vi "Host_Main.vi"() -> ()   [LabVIEW 2019]
uses:
  <vilib>/vision/NI_Vision_Development_Module.lvlib
panel:
  in  "stop":bool
  out "HeartBeatSignal":bool
  out "ZMP_Y-Axis_Position(mm)":dbl format="%.1f"
  out "XY Graph":cluster{dbl[], dbl[]}[](graph)
  out "ZMP_X-Axis_Position(mm)":dbl format="%.1f"
  in  "Ladeer_Mass(Kg)":dbl=1000.0
  in  "Ladeer_Mass_Point(mm)":dbl=1000.0
  in  "Load(Kg)":dbl=100.0
  in  "Outrigger_Front_Position(mm)":dbl=1500.0
  in  "Outrigger_Rear_Position(mm)":dbl=100.0
  in  "Outrigger_RR_Length(mm)":dbl=300.0
  in  "Outrigger_RL_Length(mm)":dbl=-300.0
  in  "Outrigger_FR_Length(mm)":dbl=500.0
  in  "Outrigger_FL_Length(mm)":dbl=-500.0
  in  "Vehicle_Mass(Kg)":dbl
  in  "Boom_Rising_Angle(Degree)":dbl
  in  "Boom_Rotation_Angle(Degree)":dbl
  # "Aerial Ladder Truck Monitoring Program"
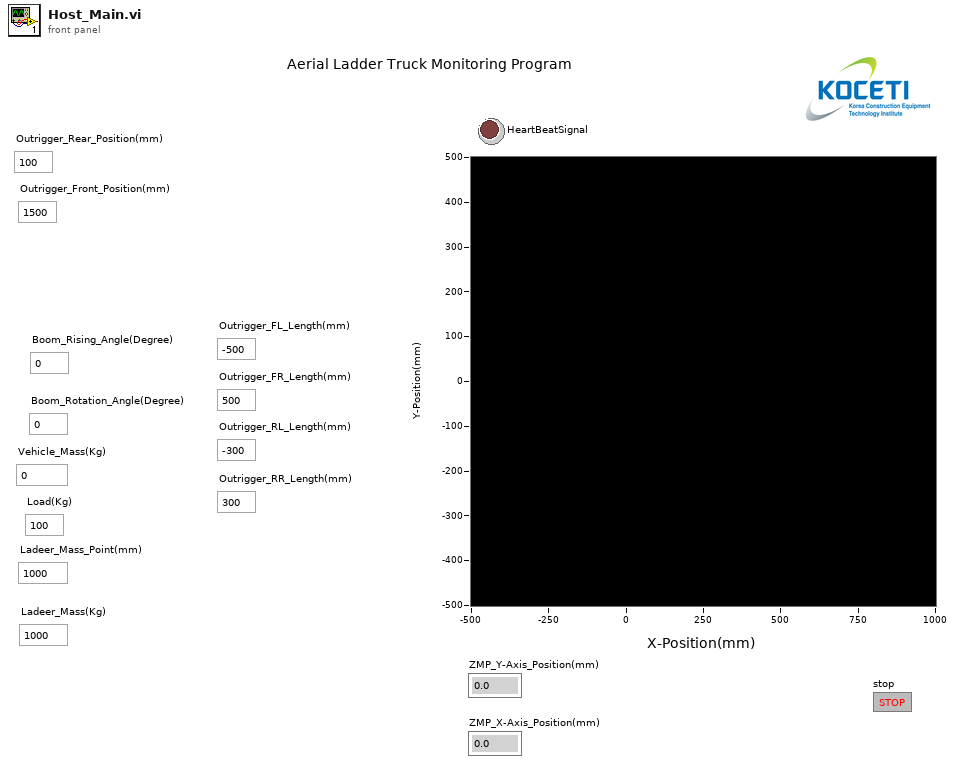
[diagram p1: front panel]
types:
  T1 = cluster{"Red or Hue value":u8, "Green or Sat value":u8, "Blue or Luma or Val or Inten value":u8}
  T2 = typedef "Image Type" = u32
  T3 = typedef "IMAQ Image.ctl" = refnum<image>
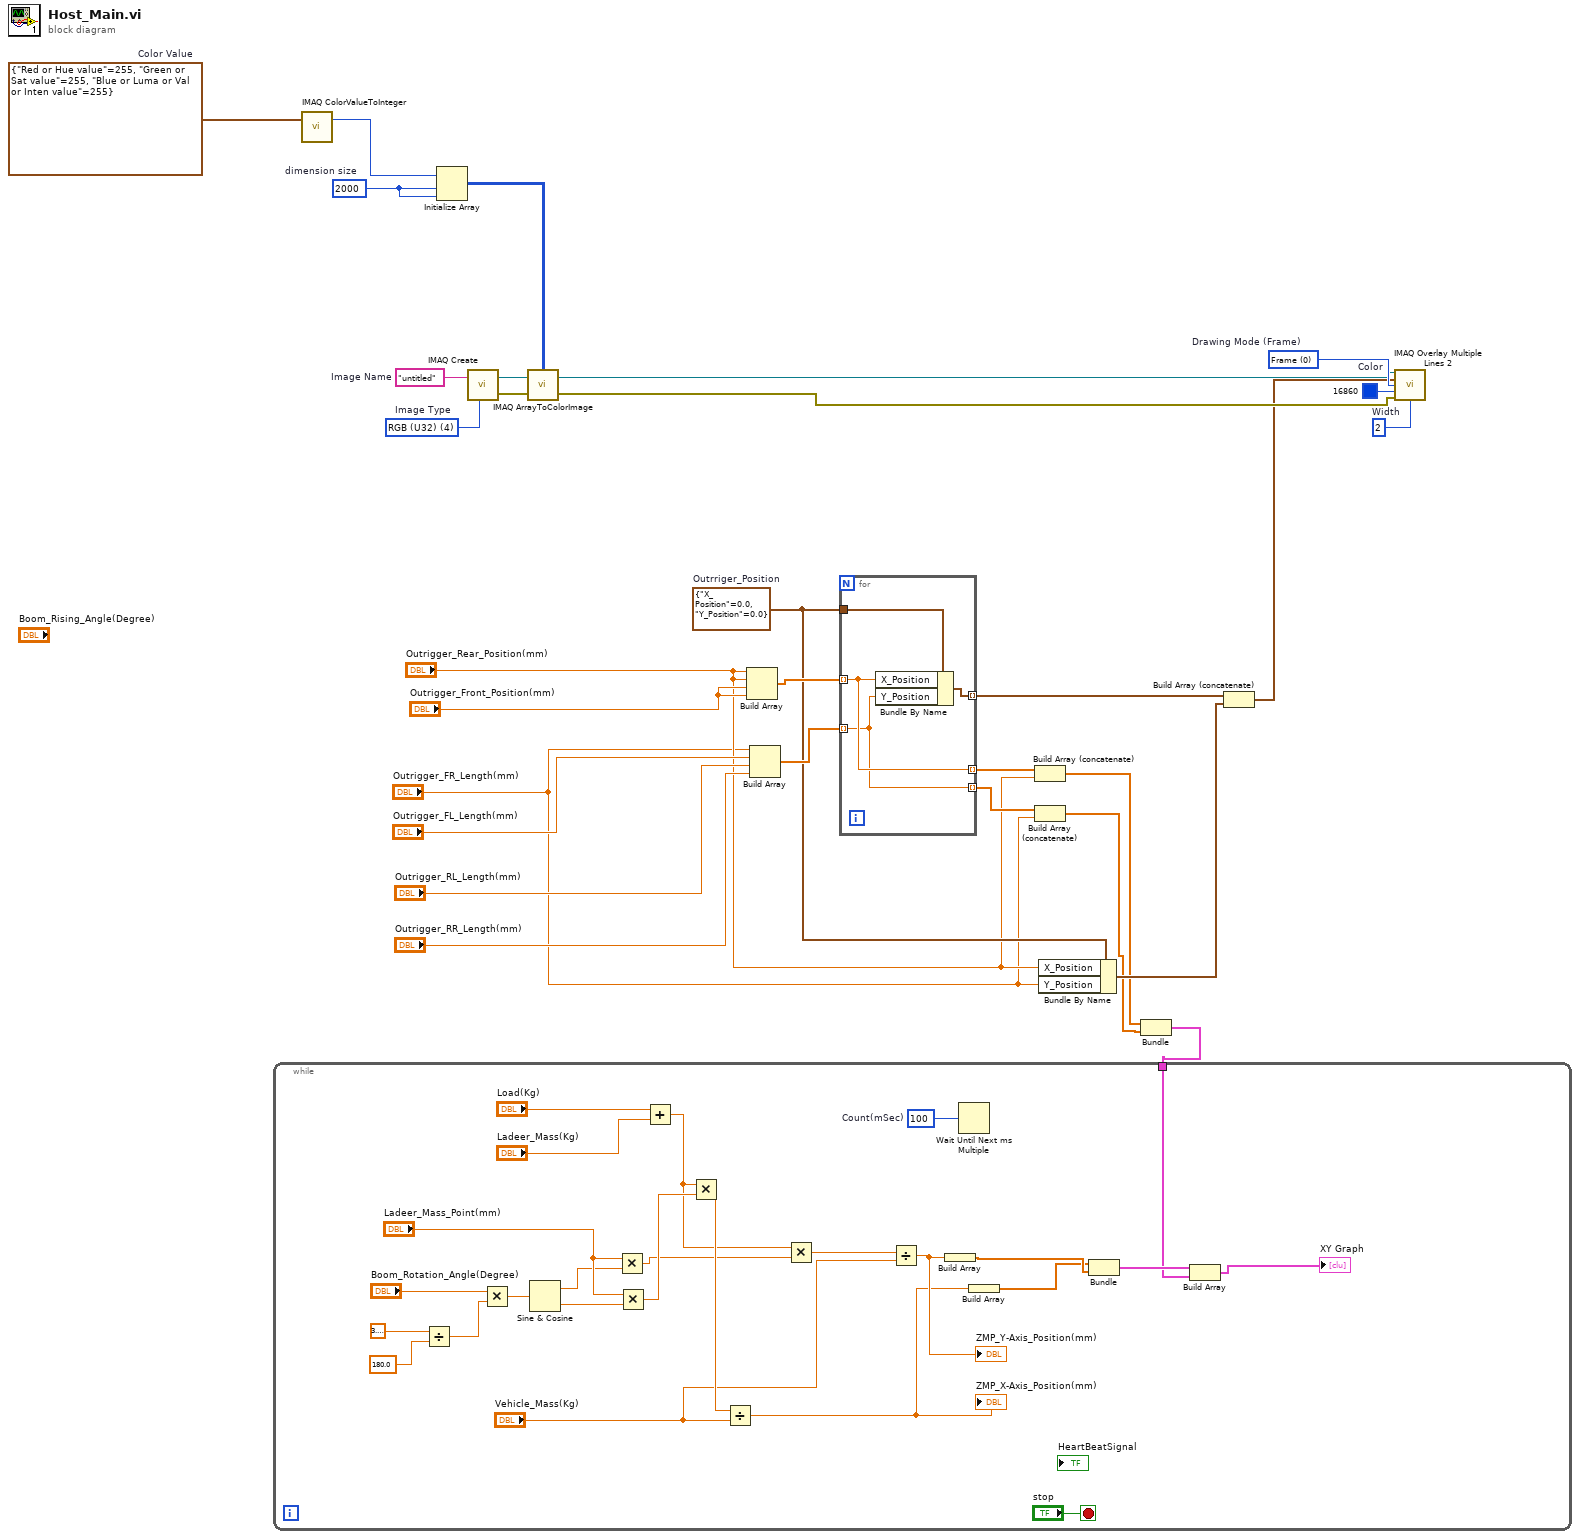
[diagram p0: block diagram]
diagram:
  w14 = 2000  # dimension size
  w18 = T1 {"Red or Hue value"=255, "Green or Sat value"=255, "Blue or Luma or Val or Inten value"=255}  # Color Value
  w20 = u32 2  # Width
  w21 = u32 0 items=["Frame", "Fill"]  # Drawing Mode (Frame)
  w22 = T2 4 items=["Grayscale (U8)", "Grayscale (I16)", "Grayscale (SGL)", "Complex (CSG)", "RGB (U32)", "HSL (U32)", "RGB (U64)", "Grayscale (U16)"]  # Image Type
  w23 = "untitled"  # Image Name
  w24 = u32 16860  # Color
  w11 = cluster{"X_Position":dbl, "Y_Position":dbl} {"X_Position"=0.0, "Y_Position"=0.0}  # Outrriger_Position
  n1 = call "IMAQ ColorValueToInteger"("Color Value"=w18) -> ("U32 value"=w16:u32)  [unwired: 4 in, 3 out]
  n2 = Initialize Array "Initialize Array"(w16, w14, w14) -> (w15:u32[][])
  n3 = call "IMAQ Create"("Image Name"=w23, "Image Type"=w22) -> ("New Image"=w19:T3, "error out"=w10:errorcluster)  [unwired: 3 in]
  n4 = call "IMAQ ArrayToColorImage"("Image Pixels (U32)"=w15, "Image"=w19, "error in (no error)"=w10) -> ("Image Out"=w17:T3, "error out"=w9:errorcluster)  [unwired: 2 in]
  n5 = Build Array("Outrigger_Rear_Position(mm)", "Outrigger_Rear_Position(mm)", "Outrigger_Front_Position(mm)", "Outrigger_Front_Position(mm)") -> (w30:dbl[])
  n6 = Build Array("Outrigger_FR_Length(mm)", "Outrigger_FL_Length(mm)", "Outrigger_RL_Length(mm)", "Outrigger_RR_Length(mm)") -> (w29:dbl[])
  n7 = for {
    tunnel: w30 -> [w32] mode=indexing
    tunnel: w11 -> [w34]
    tunnel: w29 -> [w31] mode=indexing
    tunnel: [w33] -> w25 mode=indexing
    tunnel: [w32] -> w8 mode=indexing
    tunnel: [w31] -> w7 mode=indexing
    n8 = Bundle By Name(cluster=w34, "X_Position"=w32, "Y_Position"=w31) -> (w33:cluster{"X_Position":dbl, "Y_Position":dbl})
  }
  n9 = Build Array (concatenate)(w8, "Outrigger_Rear_Position(mm)") -> (w4:dbl[])
  n10 = Build Array (concatenate)(w7, "Outrigger_FR_Length(mm)") -> (w3:dbl[])
  n11 = Bundle By Name(cluster=w11, "X_Position"="Outrigger_Rear_Position(mm)", "Y_Position"="Outrigger_FR_Length(mm)") -> (w12:cluster{"X_Position":dbl, "Y_Position":dbl})
  n12 = Bundle(w4, w3) -> (w2:cluster{dbl[], dbl[]})  [unwired: 1 in]
  n13 = while {
    tunnel: w2 -> [w36]
    stop <- "stop" stop-if-true
    w49 = u32 100  # Count(mSec)
    n14 = Divide(x=3.141592653589793, y=180.0) -> (x/y=w56:dbl)
    n15 = Multiply(x="Boom_Rotation_Angle(Degree)", y=w56) -> (x*y=w57:dbl)
    n16 = Sine & Cosine(0:w57) -> (1:w46:dbl, 2:w51:dbl)
    n17 = Multiply(x="Ladeer_Mass_Point(mm)", y=w46) -> (x*y=w45:dbl)
    n18 = Multiply(x="Ladeer_Mass_Point(mm)", y=w51) -> (x*y=w50:dbl)
    n19 = Add(x="Load(Kg)", y="Ladeer_Mass(Kg)") -> (x+y=w48:dbl)
    n20 = Multiply(x=w48, y=w50) -> (x*y=w53:dbl)
    n21 = Divide(x=w53, y="Vehicle_Mass(Kg)") -> (x/y=w41:dbl)
    "ZMP_X-Axis_Position(mm)" <- w41
    n22 = Multiply(x=w48, y=w45) -> (x*y=w44:dbl)
    n23 = Divide(x=w44, y="Vehicle_Mass(Kg)") -> (x/y=w42:dbl)
    "ZMP_Y-Axis_Position(mm)" <- w42
    n24 = Build Array(w42) -> (w40:dbl[])
    n25 = Wait Until Next ms Multiple(millisecond multiple=w49) -> ()  [unwired: 1 out]
    n26 = Build Array(w41) -> (w39:dbl[])
    n27 = Bundle(w39, w40) -> (w38:cluster{dbl[], dbl[]})  [unwired: 1 in]
    n28 = Build Array(w38, w36) -> (→"XY Graph":cluster{dbl[], dbl[]}[])
  }
  n29 = Build Array (concatenate)(w25, w12) -> (w1:cluster{"X_Position":dbl, "Y_Position":dbl}[])
  n30 = call "IMAQ Overlay Multiple Lines 2"("Image"=w17, "Line End Points"=w1, "Drawing Mode (Frame)"=w21, "Color"=w24, "error in (no error)"=w9, "Width"=w20) -> ()  [unwired: 8 in, 2 out]
